vi "Receive Value Change Event.vi"(8 "error in (no error)":errorcluster, 10 "ValueChangeMsg":refnum<class "ValueChangeMsg.lvclass">, 11 "Main ViewManager In":refnum<class "Main ViewManager.lvclass">) -> (0 "error out":errorcluster, 3 "Main ViewManager Out":refnum<class "Main ViewManager.lvclass">)   [LabVIEW 2019, in "Main ViewManager.lvclass"]
doc: "<License>\nCopyright © 2017 Composed Systems, LLC | All rights reserved\nwww.composed.io\n\nAuthor: Ethan Stern <ethan.stern@composed.io>\n\nThis software is provided \"AS IS\" WITHOUT WARRANTIES, either express or implied, AND IS FOR EDUCATIONAL PURPOSES ONLY.\n</License>"
uses:
  <vilib>/gpm_packages/@cs/Car-wash/Source/Main ViewManager/Main ViewManager/Main ViewManager.lvclass
  <vilib>/gpm_packages/@cs/mva-viewable/Source/IViewManager/IViewManager/IViewManager.lvclass
  <vilib>/gpm_packages/@cs/mva-viewable/Source/ActorEvents/IEventAggregator Messages/ValueChangeMsg/ValueChangeMsg.lvclass
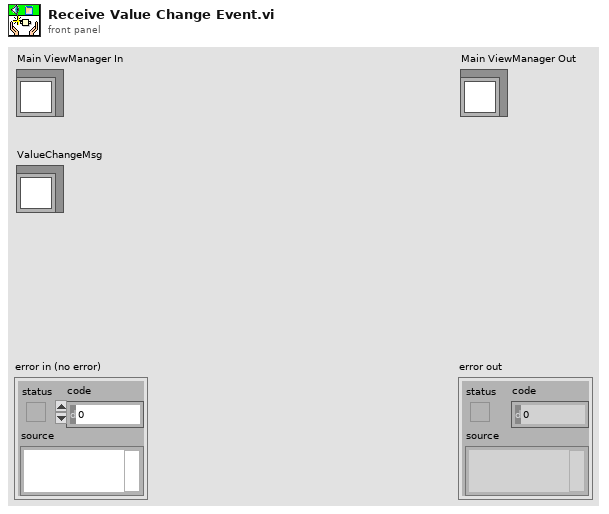
[diagram p1: front panel]
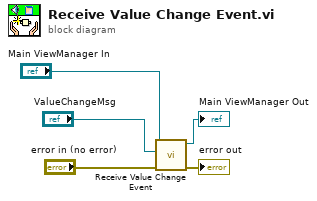
[diagram p0: block diagram]
diagram:
  n1 = call-parent "Receive Value Change Event.vi"("error in (no error)"="error in (no error)", "ValueChangeMsg"="ValueChangeMsg", "IViewable In"="Main ViewManager In") -> ("error out"=→"error out":errorcluster, "IViewable Out"=→"Main ViewManager Out":refnum<class "Main ViewManager.lvclass">)  [unwired: 7 in]
